vi "Autonomous Independent.vi"() -> ()   [LabVIEW 2012]
doc: "This VI is called when autonomous begins, and will automatically be terminated when autonomous ends. You can carry out timed or sensor driven robot movement independently without needing to return to the caller."
uses:
  <vilib>/Rock Robotics/WPI/Relay/WPI_RelayValue.ctl
  <vilib>/Rock Robotics/WPI/RobotDrive/WPI_RobotDriveGetSetRefNum.vi
  Robot Global Data.vi
panel:
  out "Shooter Speed":T1(ring)
  out "Stop Drive":bool
  out "DT Output":enum16{"Off", "Up", "Down"}(ring)=enum."Down"
  out "BAD Up":bool
  out "DAD Output":T2
  out "Shift Low":bool
  out "Feeder Happy":bool
  out "Auton Done":bool
  out "Shooter Happy":bool
  out "Shoot!":bool
  out "Loop Rate (Hz)":dbl
  out "Delay Switch":u32
  out "Seccond Switch":u32
  out "First Switch":u32
  # "Be sure to right-click and choose Data Operations>>Make Current Value default if you want to save the array values with the VI"
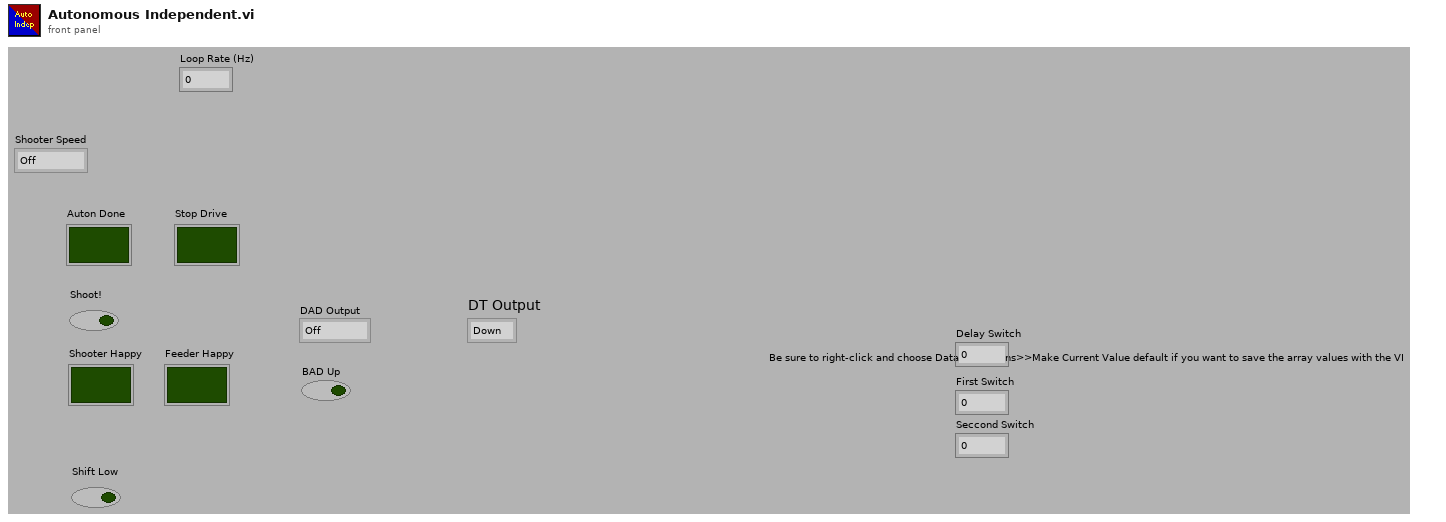
[diagram p1: front panel]
types:
  T1 = enum16{"Off", "Close Pyramid 3pt", "Far Pyramid 3pt", "Feeder Shot"}
  T2 = typedef "WPI_RelayValue.ctl" = enum16{"Off", "On", "Forward", "Reverse"}
  T3 = typedef "WPI_RobotDriveDevRef.ctl" = cluster{"DevStatus":errorcluster, "Motors[]":T4[], "Square Inputs":bool, "Max Output":dbl, "Isochronous":bool}
  T4 = typedef "WPI_MotorControlDeviceRef.ctl" = cluster{"DeviceStatus":errorcluster, "Type":enum16{"PWM", "CAN"}, "PWM":cluster{"Digital Module":T5, "PWM Channel":T6, "DeadBand":T7}, "CAN":cluster{"Device Number":u8, "Control Mode":T8, "Semaphore":T9, "Max Vout":dbl}, "Invert":bool, "TransformRef":T10, "InvTransformRef":T10}
  T5 = typedef "FPGA_TypedefDigitalModule.ctl" = enum16{"Digital Module 1", "Digital Module 2"}
  T6 = typedef "FPGA_DIOPWMChannel.ctl" = enum8{"PWM 1", "PWM 2", "PWM 3", "PWM 4", "PWM 5", "PWM 6", "PWM 7", "PWM 8", "PWM 9", "PWM 10", "Invalid"}
  T7 = typedef "WPI_PWMDeadband.ctl" = cluster{"Name":string, "maxPositivePwm":i32, "minPositivePwm":i32, "centerPwm":i32, "maxNegativePwm":i32, "minNegativePwm":i32, "angularRange":u16}
  T8 = typedef "WPI_CANJaguar_ControlMode.ctl" = enum8{"Percent VBus", "Current", "Speed", "Position", "Voltage"}
  T9 = typedef "Semaphore RefNum" = refnum<k1>
  T10 = typedef "WPI_PWMTransform_ConPane.ctl" = refnum<vi>
  T11 = typedef "WPI_GyroDevRef.ctl" = cluster{"DevStatus":errorcluster, "Analog Module":T12, "Analog Channel":T13, "Offset":dbl, "Gain (VoltsPerDegree/Second)":dbl}
  T12 = typedef "FPGA_TypedefAnalogModule.ctl" = enum16{"Analog Module 1", "Analog Module 2"}
  T13 = typedef "FPGA_AIChannel.ctl" = enum8{"AI 1", "AI 2", "AI 3", "AI 4", "AI 5", "AI 6", "AI 7", "AI 8", "Invalid"}
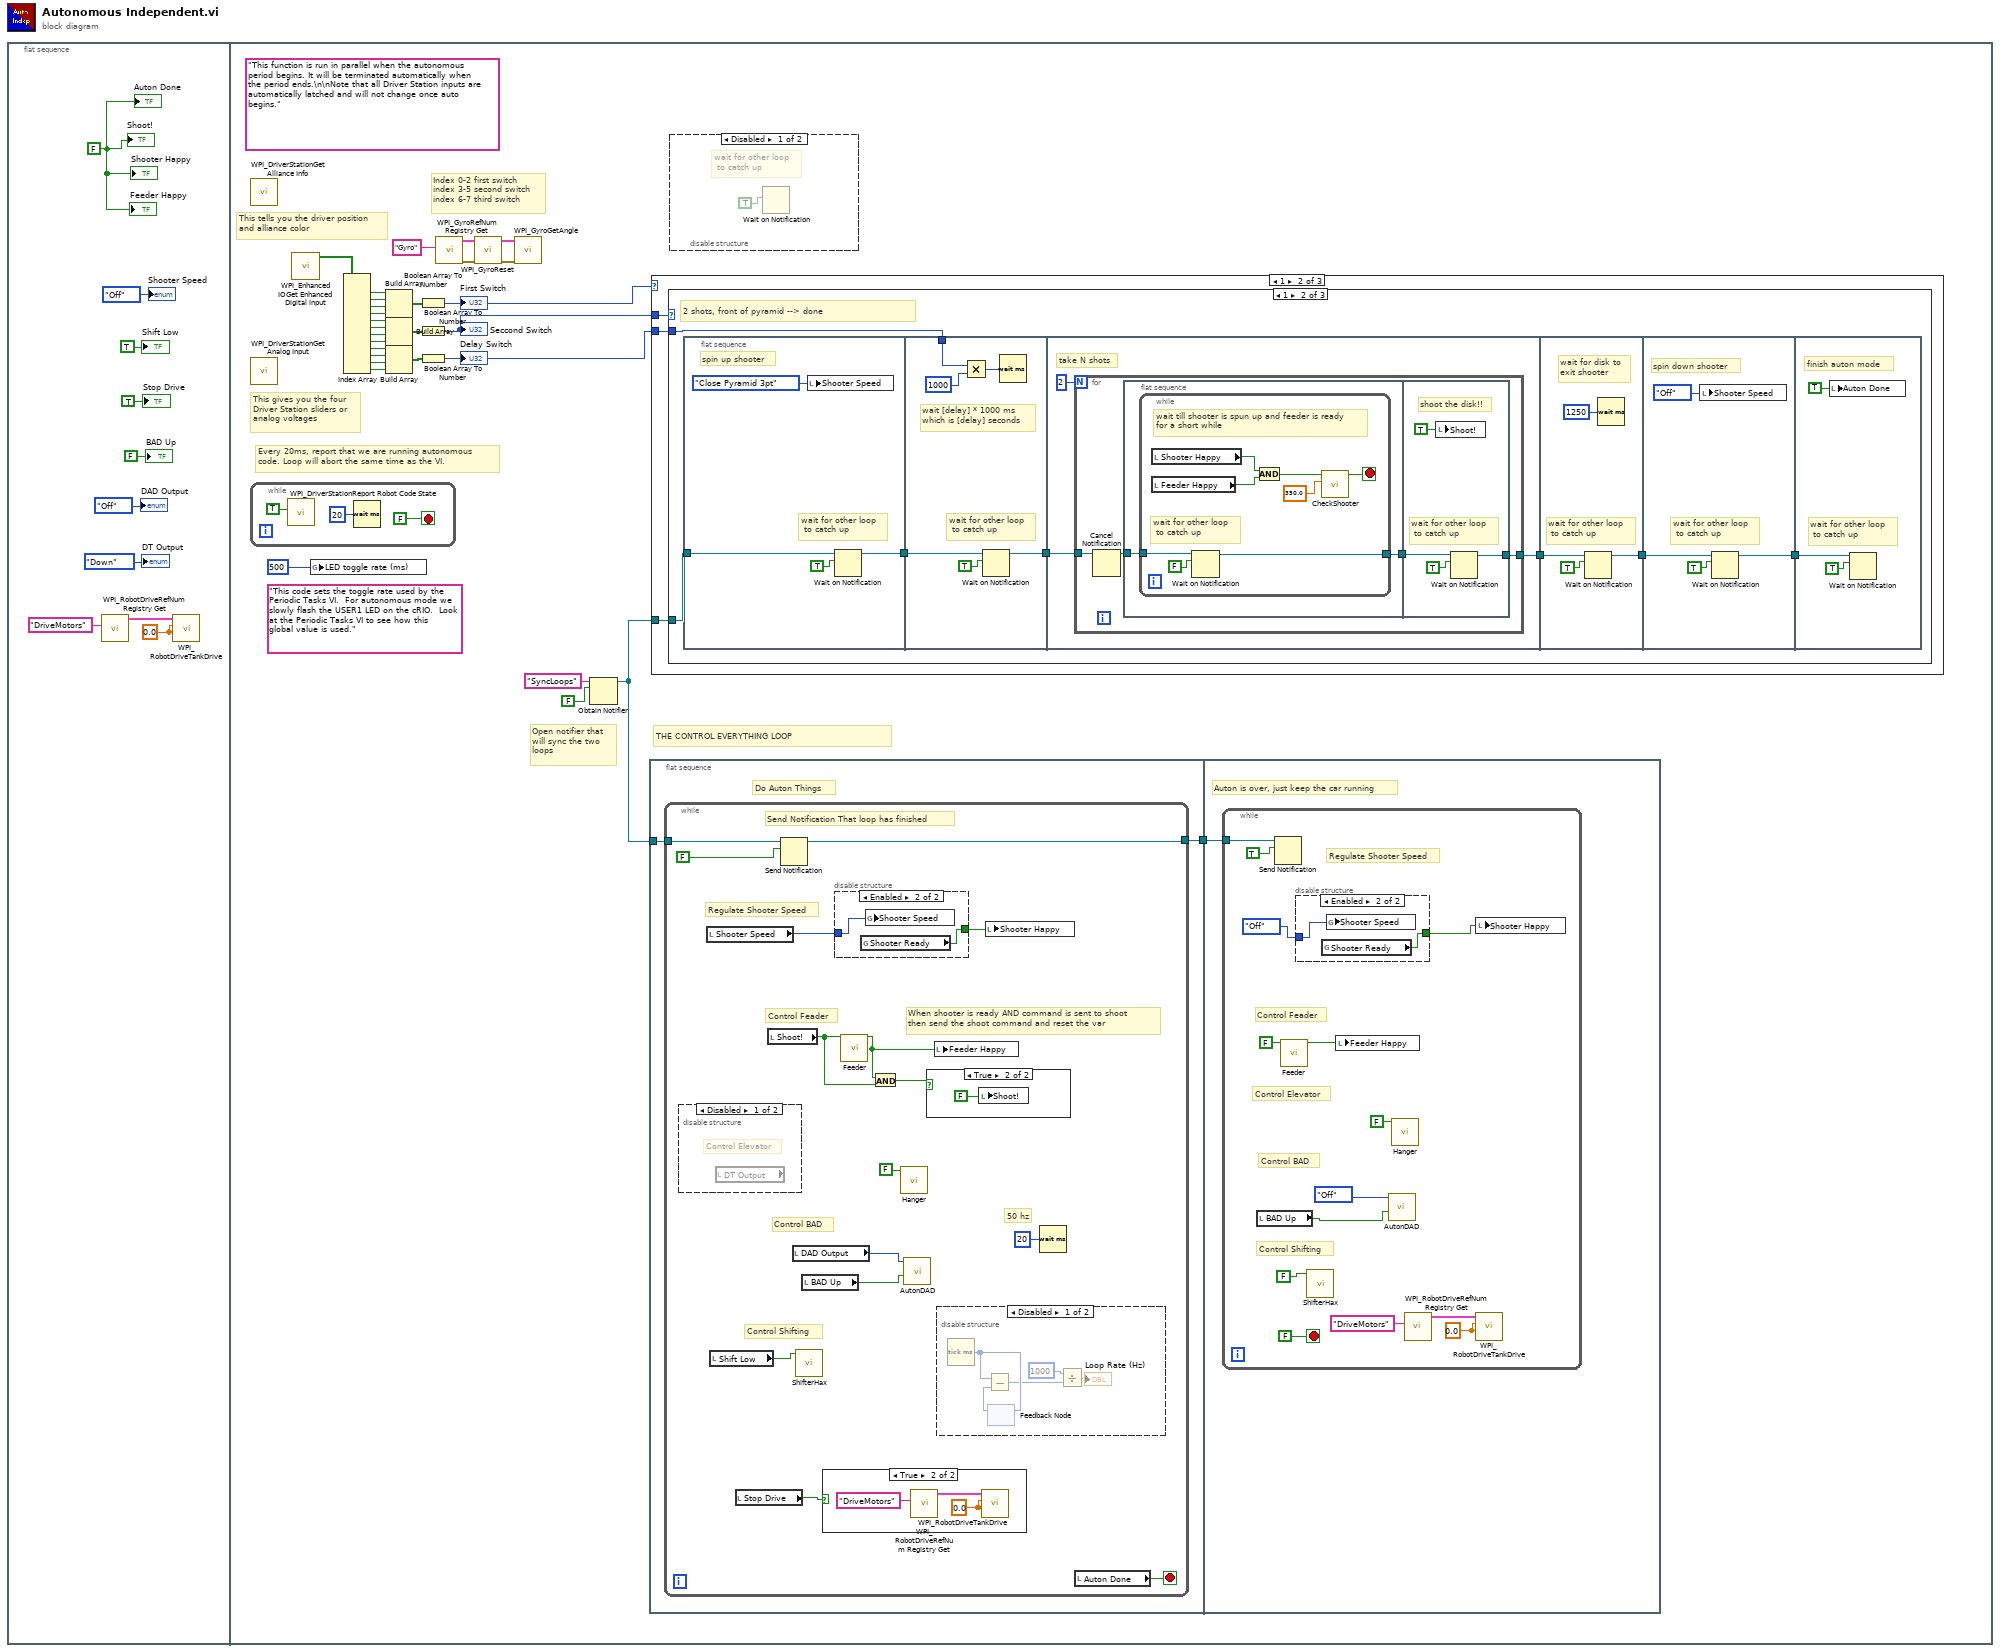
[diagram p0: block diagram]
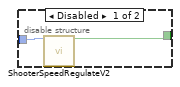
[diagram p3: hidden frame]
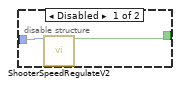
[diagram p8: hidden frame]
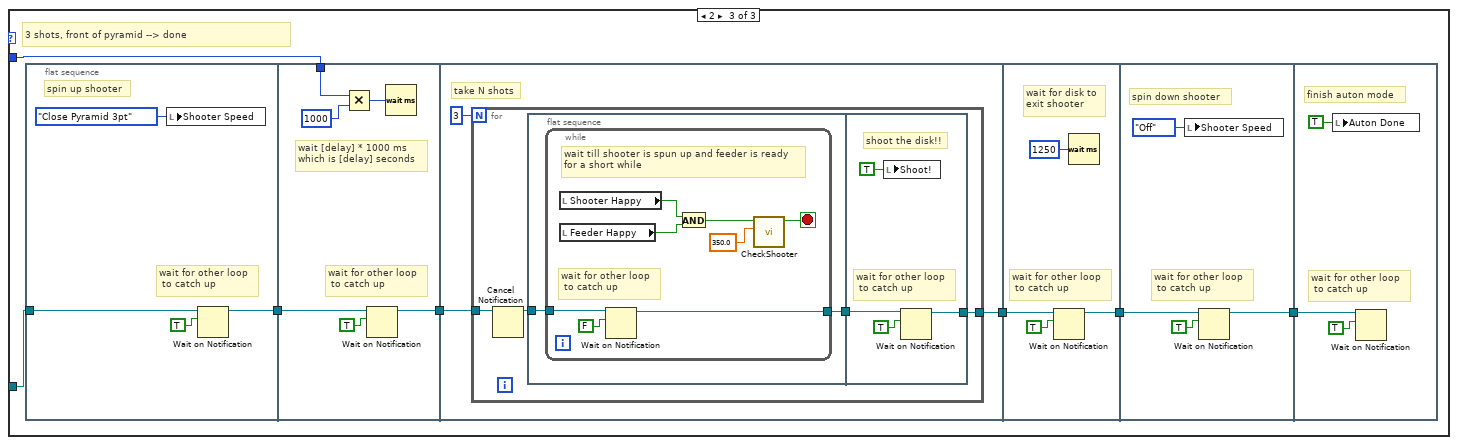
[diagram p11: hidden frame]
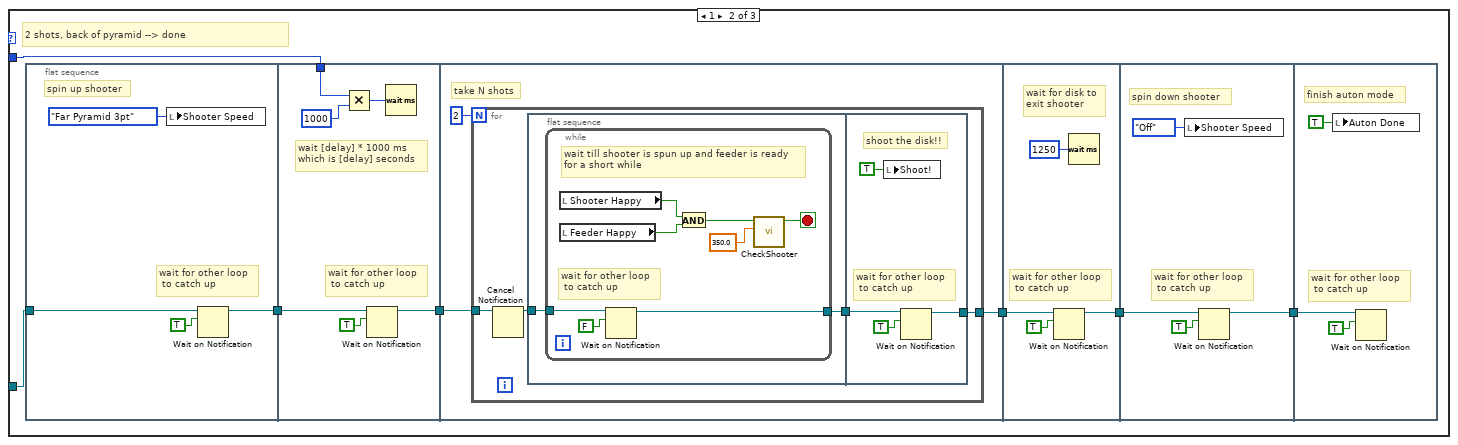
[diagram p13: hidden frame]
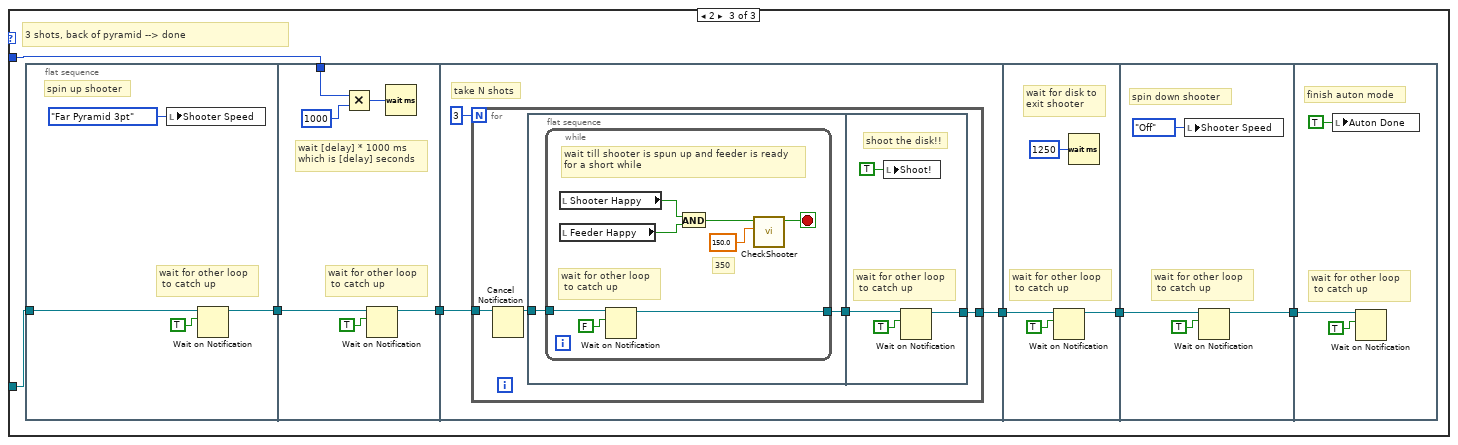
[diagram p14: hidden frame]
diagram:
  n1 = flat-sequence {
    frame #0 {
      w3 = 0.0 ("Left axis value")
      w10 = FALSE
      n2 = call <vilib>:"WPI_RobotDriveRefNum Registry Get.vi"("refnum name"="DriveMotors") -> ("RobotDriveDevRef"=w5:T3)  [unwired: 1 in, 9 out]
      n3 = call <vilib>:"WPI_RobotDriveTankDrive.vi"("Right axis value"=w3, "Left axis value"=w3, "RobotDriveDevRef"=w5) -> ()  [unwired: 6 in, 3 out]
      "Feeder Happy" <- w10
      "Shift Low" <- TRUE ("Shift Low")
      "DAD Output" <- WPI_RelayValue."Off" ("DAD Output")
      "BAD Up" <- FALSE ("BAD Up")
      "Stop Drive" <- TRUE ("Stop Drive")
      "Shoot!" <- w10
      "Shooter Happy" <- w10
      "Auton Done" <- w10
      "DT Output" <- enum16{"Off", "Up", "Down"}."Down" ("DT Output")
      "Shooter Speed" <- T1."Off" ("Shooter Speed")
    }
    frame #1 {
      (unwired) "This code sets the toggle rate used by the Periodic Tasks VI.  For autonomous mode we slowly flash the USER1 LED on the cRIO.  Look at the Periodic Tasks VI to see how this global value is used."
      (unwired) "This function is run in parallel when the autonomous period begins. It will be terminated automatically when the period ends.\n\nNote that all Driver Station inputs are automatically latched and will not change once auto begins."
      # "THE CONTROL EVERYTHING LOOP"
      # "Index 0-2 first switch\nindex 3-5 second switch\nindex 6-7 third switch"
      # "Open notifier that\nwill sync the two\nloops"
      # "Every 20ms, report that we are running autonomous\ncode. Loop will abort the same time as the VI."
      # "This tells you the driver position\nand alliance color"
      # "This gives you the four\nDriver Station sliders or\nanalog voltages"
      n4 = call <vilib>:"WPI_DriverStationGet Alliance Info.vi"() -> ()  [unwired: 12 out]
      n5 = call <vilib>:"WPI_DriverStationGet Analog Input.vi"() -> ()  [unwired: 12 out]
      n6 = while {
        stop <- FALSE stop-if-true
        n7 = call <vilib>:"WPI_DriverStationReport Robot Code State.vi"("Autonomous"=TRUE) -> ()  [unwired: 10 in, 1 out]
        n8 = Wait (ms)(milliseconds to wait=u32 20) -> ()  [unwired: 1 out]
      }
      n9 = call <vilib>:"WPI_Enhanced IOGet Enhanced Digital Input.vi"() -> ("Digital Input [1-16]"=w15:bool[])  [unwired: 10 in, 1 out]
      n10 = global write "Robot Global Data.vi" "LED toggle rate (ms)"(u32 500 ("LED ms toggle rate")) -> ()
      n11 = Index Array(array=w15) -> (element #1=w35:bool, element #2=w34:bool, element #3=w33:bool, element #4=w21:bool, element #5=w32:bool, element #6=w31:bool, element #7=w23:bool, element #8=w22:bool, element #9=w20:bool, element #10=w19:bool, element #11=w18:bool, element #12=w17:bool)  [unwired: 12 in]
      n12 = Build Array(w35, w34, w33, w21) -> (w29:bool[])
      n13 = Build Array(w32, w31, w23, w22) -> (w30:bool[])
      n14 = Build Array(w20, w19, w18, w17) -> (w16:bool[])
      n15 = Boolean Array To Number(Boolean array=w29) -> (number=w14:u32)
      "First Switch" <- w14
      n16 = Boolean Array To Number(Boolean array=w30) -> (number=w13:u32)
      "Seccond Switch" <- w13
      n17 = Boolean Array To Number(Boolean array=w16) -> (number=w11:u32)
      "Delay Switch" <- w11
      n18 = call <vilib>:"WPI_GyroRefNum Registry Get.vi"("refnum name"="Gyro") -> ("error out"=w24:errorcluster, "GyroDevRef"=w25:T11)  [unwired: 9 in]
      n19 = call <vilib>:"WPI_GyroReset.vi"("error in (no error)"=w24, "GyroDevRef"=w25) -> ("error out"=w27:errorcluster, "GyroDevRef"=w26:T11)  [unwired: 8 in]
      n20 = call <vilib>:"WPI_GyroGetAngle.vi"("error in (no error)"=w27, "GyroDevRef"=w26) -> ()  [unwired: 6 in, 4 out]
      n21 = Obtain Notifier(name (unnamed)="SyncLoops", notification data type=FALSE) -> (notifier out=w12:refnum<notifier>)  [unwired: 2 in, 2 out]
      n22 = flat-sequence {
        tunnel: w12 -> [w43]
        tunnel: [w42] -> w39
        tunnel: w39 -> [w72]
        frame #0 {
          # "Do Auton Things"
          n23 = while {
            tunnel: w43 -> [w56]
            tunnel: [w52] -> w42
            stop <- w58 stop-if-true
            # "Regulate Shooter Speed"
            # "50 hz"
            # "Control BAD"
            # "Control Shifting"
            # "When shooter is ready AND command is sent to shoot\nthen send the shoot command and reset the var"
            # "Control Feader"
            # "Send Notification That loop has finished"
            n24 = disable-structure shown="Disabled" {
              frame Disabled {
                # "Control Elevator"
                n25 = local read "DT Output"() -> ()  [unwired: 1 out]
              }
              frame Enabled {
              }
            }
            n26 = local read "Shooter Speed"() -> (w45:T1)
            n27 = local read "Shift Low"() -> (w46:bool)
            n28 = local read "Stop Drive"() -> (w50:bool)
            n29 = local read "Shoot!"() -> (w55:bool)
            n30 = Send Notification(notification=FALSE, notifier=w56) -> (notifier out=w52:refnum<notifier>)  [unwired: 1 in, 1 out]
            n31 = local read "DAD Output"() -> (w48:T2)
            n32 = call "ShifterHax.vi"("Shift low?"=w46) -> ()  [unwired: 11 in]
            n33 = local read "BAD Up"() -> (w49:bool)
            n34 = case shown="True" w50 {
              frame False {
              }
              frame True {
                w65 = 0.0 ("Left axis value")
                n35 = call <vilib>:"WPI_RobotDriveRefNum Registry Get.vi"("refnum name"="DriveMotors") -> ("RobotDriveDevRef"=w63:T3)  [unwired: 1 in, 9 out]
                n36 = call <vilib>:"WPI_RobotDriveTankDrive.vi"("Right axis value"=w65, "Left axis value"=w65, "RobotDriveDevRef"=w63) -> ()  [unwired: 6 in, 3 out]
              }
            }
            n37 = disable-structure shown="Enabled" {
              disable-tunnel: [w60 w61] -> w47
              disable-tunnel: w45 -> [w59 w62]
              frame Disabled {
                n38 = call "ShooterSpeedRegulateV2.vi"("Shooter Speed"=w59) -> ("ALL GOOD"=w60:bool)  [unwired: 13 in, 1 out]
              }
              frame Enabled {
                n39 = global read "Robot Global Data.vi" "Shooter Ready"() -> (w61:bool)
                n40 = global write "Robot Global Data.vi" "Shooter Speed"(w62) -> ()
              }
            }
            n41 = call "Feeder.vi"("SHOOT Button"=w55) -> ("Ready To Shoot?"=w53:bool)  [unwired: 10 in]
            n42 = And(x=w53, y=w55) -> (x .and. y?=w54:bool)
            n43 = call "Hanger.vi"("Hanger Up"=FALSE) -> ()  [unwired: 10 in, 1 out]
            n44 = call "AutonDAD.vi"("BAD UP"=w49, "BAD Output"=w48) -> ()  [unwired: 10 in]
            n45 = case shown="True" w54 {
              frame False {
              }
              frame True {
                n46 = local write "Shoot!"(FALSE) -> ()
              }
            }
            n47 = local write "Feeder Happy"(w53) -> ()
            n48 = disable-structure shown="Disabled" {
              frame Disabled {
                n49 = Tick Count (ms)() -> (millisecond timer value=w70:u32)
                n50 = feedback #1() -> (w69:u32)  [unwired: 1 in]
                n51 = Subtract(x=w70, y=w69) -> (x-y=w67:u32)
                n52 = feedback-in #1(w70) -> ()
                n53 = Divide(x=1000, y=w67) -> (x/y=→"Loop Rate (Hz)":dbl)
              }
              frame Enabled {
              }
            }
            n54 = local write "Shooter Happy"(w47) -> ()
            n55 = Wait (ms)(milliseconds to wait=u32 20) -> ()  [unwired: 1 out]
            n56 = local read "Auton Done"() -> (w58:bool)
          }
        }
        frame #1 {
          # "Auton is over, just keep the car running"
          n57 = while {
            tunnel: w72 -> [w76]
            stop <- FALSE stop-if-true
            w81 = 0.0 ("Left axis value")
            # "Regulate Shooter Speed"
            # "Control BAD"
            # "Control Shifting"
            # "Control Elevator"
            # "Control Feader"
            n58 = local read "BAD Up"() -> (w79:bool)
            n59 = Send Notification(notification=TRUE, notifier=w76) -> ()  [unwired: 1 in, 2 out]
            n60 = call "Feeder.vi"("SHOOT Button"=FALSE) -> ("Ready To Shoot?"=w85:bool)  [unwired: 10 in]
            n61 = disable-structure shown="Enabled" {
              disable-tunnel: [w88 w89] -> w73
              disable-tunnel: T1."Off" ("Shooter Speed") -> [w87 w90]
              frame Disabled {
                n62 = call "ShooterSpeedRegulateV2.vi"("Shooter Speed"=w87) -> ("ALL GOOD"=w88:bool)  [unwired: 13 in, 1 out]
              }
              frame Enabled {
                n63 = global read "Robot Global Data.vi" "Shooter Ready"() -> (w89:bool)
                n64 = global write "Robot Global Data.vi" "Shooter Speed"(w90) -> ()
              }
            }
            n65 = call "ShifterHax.vi"("Shift low?"=FALSE ("Shifting Button")) -> ()  [unwired: 11 in]
            n66 = local write "Feeder Happy"(w85) -> ()
            n67 = call "AutonDAD.vi"("BAD UP"=w79, "BAD Output"=WPI_RelayValue."Off") -> ()  [unwired: 10 in]
            n68 = call "Hanger.vi"("Hanger Up"=FALSE) -> ()  [unwired: 10 in, 1 out]
            n69 = call <vilib>:"WPI_RobotDriveRefNum Registry Get.vi"("refnum name"="DriveMotors") -> ("RobotDriveDevRef"=w83:T3)  [unwired: 1 in, 9 out]
            n70 = call <vilib>:"WPI_RobotDriveTankDrive.vi"("Right axis value"=w81, "Left axis value"=w81, "RobotDriveDevRef"=w83) -> ()  [unwired: 6 in, 3 out]
            n71 = local write "Shooter Happy"(w73) -> ()
          }
        }
      }
      n72 = case shown="1" w14 {
        tunnel: w13 -> [_ w93 w194]
        tunnel: w12 -> [_ w92 w193]
        tunnel: w11 -> [_ w91 w192]
        frame 0, Default {
          # "do nothing"
        }
        frame 1 {
          n73 = case shown="1" w93 {
            tunnel: w92 -> [_ w97 w146]
            tunnel: w91 -> [_ w100 w149]
            frame 0, Default {
              # "do nothing"
            }
            frame 1 {
              # "2 shots, front of pyramid --> done"
              n74 = flat-sequence {
                tunnel: [w103] -> w99
                tunnel: w97 -> [w102]
                tunnel: w100 -> [w108]
                tunnel: w99 -> [w106]
                tunnel: [w105] -> w98
                tunnel: w98 -> [w112]
                tunnel: [w111] -> w94
                tunnel: [w133] -> w95
                tunnel: w94 -> [w132]
                tunnel: [w138] -> w96
                tunnel: w95 -> [w137]
                tunnel: w96 -> [w140]
                frame #0 {
                  # "wait for other loop\n to catch up"
                  # "spin up shooter"
                  n75 = local write "Shooter Speed"(T1."Close Pyramid 3pt" ("Shooter Speed")) -> ()
                  n76 = Wait on Notification(notifier=w102, ignore previous (F)=TRUE) -> (notifier out=w103:refnum<notifier>)  [unwired: 2 in, 3 out]
                }
                frame #1 {
                  # "wait for other loop\n to catch up"
                  # "wait [delay] * 1000 ms\nwhich is [delay] seconds"
                  n77 = Multiply(x=w108, y=1000) -> (x*y=w110:u32)
                  n78 = Wait on Notification(notifier=w106, ignore previous (F)=TRUE) -> (notifier out=w105:refnum<notifier>)  [unwired: 2 in, 3 out]
                  n79 = Wait (ms)(milliseconds to wait=w110) -> ()  [unwired: 1 out]
                }
                frame #2 {
                  # "take N shots"
                  n80 = for {
                    N: 2 -> [_]
                    tunnel: w112 -> [w116]
                    tunnel: [w114] -> w111
                    n81 = Cancel Notification(0:w116) -> (8:w117:refnum<notifier>)  [unwired: 1 in, 2 out]
                    n82 = flat-sequence {
                      tunnel: w117 -> [w119]
                      tunnel: [w118] -> w115
                      tunnel: w115 -> [w129]
                      tunnel: [w128] -> w114
                      frame #0 {
                        n83 = while {
                          tunnel: w119 -> [w121]
                          tunnel: [w120] -> w118
                          stop <- w123 stop-if-true
                          # "wait for other loop\n to catch up"
                          # "wait till shooter is spun up and feeder is ready\nfor a short while"
                          n84 = local read "Shooter Happy"() -> (w126:bool)
                          n85 = local read "Feeder Happy"() -> (w125:bool)
                          n86 = Wait on Notification(notifier=w121, ignore previous (F)=FALSE) -> (notifier out=w120:refnum<notifier>)  [unwired: 2 in, 3 out]
                          n87 = And(x=w126, y=w125) -> (x .and. y?=w124:bool)
                          n88 = call "CheckShooter.vi"("Time for happy (ms)"=350.0, "Shooter Good?"=w124) -> ("Good to shoot"=w123:bool)  [unwired: 9 in]
                        }
                      }
                      frame #1 {
                        # "wait for other loop\n to catch up"
                        # "shoot the disk!!"
                        n89 = local write "Shoot!"(TRUE ("Shoot!")) -> ()
                        n90 = Wait on Notification(notifier=w129, ignore previous (F)=TRUE) -> (notifier out=w128:refnum<notifier>)  [unwired: 2 in, 3 out]
                      }
                    }
                  }
                }
                frame #3 {
                  # "wait for other loop\n to catch up"
                  # "wait for disk to\nexit shooter"
                  n91 = Wait on Notification(notifier=w132, ignore previous (F)=TRUE) -> (notifier out=w133:refnum<notifier>)  [unwired: 2 in, 3 out]
                  n92 = Wait (ms)(milliseconds to wait=u32 1250) -> ()  [unwired: 1 out]
                }
                frame #4 {
                  # "wait for other loop\n to catch up"
                  # "spin down shooter"
                  n93 = local write "Shooter Speed"(T1."Off" ("Shooter Speed")) -> ()
                  n94 = Wait on Notification(notifier=w137, ignore previous (F)=TRUE) -> (notifier out=w138:refnum<notifier>)  [unwired: 2 in, 3 out]
                }
                frame #5 {
                  # "wait for other loop\n to catch up"
                  # "finish auton mode"
                  n95 = local write "Auton Done"(TRUE ("Auton Done")) -> ()
                  n96 = Wait on Notification(notifier=w140, ignore previous (F)=TRUE) -> ()  [unwired: 2 in, 4 out]
                }
              }
            }
            frame 2 {
              # "3 shots, front of pyramid --> done"
              n97 = flat-sequence {
                tunnel: [w152] -> w148
                tunnel: w146 -> [w151]
                tunnel: w149 -> [w157]
                tunnel: w148 -> [w155]
                tunnel: [w154] -> w147
                tunnel: w147 -> [w161]
                tunnel: [w160] -> w143
                tunnel: [w182] -> w144
                tunnel: w143 -> [w181]
                tunnel: [w187] -> w145
                tunnel: w144 -> [w186]
                tunnel: w145 -> [w189]
                frame #0 {
                  # "wait for other loop\n to catch up"
                  # "spin up shooter"
                  n98 = local write "Shooter Speed"(T1."Close Pyramid 3pt" ("Shooter Speed")) -> ()
                  n99 = Wait on Notification(notifier=w151, ignore previous (F)=TRUE) -> (notifier out=w152:refnum<notifier>)  [unwired: 2 in, 3 out]
                }
                frame #1 {
                  # "wait for other loop\n to catch up"
                  # "wait [delay] * 1000 ms\nwhich is [delay] seconds"
                  n100 = Multiply(x=w157, y=1000) -> (x*y=w159:u32)
                  n101 = Wait on Notification(notifier=w155, ignore previous (F)=TRUE) -> (notifier out=w154:refnum<notifier>)  [unwired: 2 in, 3 out]
                  n102 = Wait (ms)(milliseconds to wait=w159) -> ()  [unwired: 1 out]
                }
                frame #2 {
                  # "take N shots"
                  n103 = for {
                    N: 3 -> [_]
                    tunnel: w161 -> [w165]
                    tunnel: [w163] -> w160
                    n104 = Cancel Notification(0:w165) -> (8:w166:refnum<notifier>)  [unwired: 1 in, 2 out]
                    n105 = flat-sequence {
                      tunnel: w166 -> [w168]
                      tunnel: [w167] -> w164
                      tunnel: w164 -> [w178]
                      tunnel: [w177] -> w163
                      frame #0 {
                        n106 = while {
                          tunnel: w168 -> [w170]
                          tunnel: [w169] -> w167
                          stop <- w172 stop-if-true
                          # "wait for other loop\n to catch up"
                          # "wait till shooter is spun up and feeder is ready\nfor a short while"
                          n107 = local read "Shooter Happy"() -> (w175:bool)
                          n108 = local read "Feeder Happy"() -> (w174:bool)
                          n109 = Wait on Notification(notifier=w170, ignore previous (F)=FALSE) -> (notifier out=w169:refnum<notifier>)  [unwired: 2 in, 3 out]
                          n110 = And(x=w175, y=w174) -> (x .and. y?=w173:bool)
                          n111 = call "CheckShooter.vi"("Time for happy (ms)"=350.0, "Shooter Good?"=w173) -> ("Good to shoot"=w172:bool)  [unwired: 9 in]
                        }
                      }
                      frame #1 {
                        # "wait for other loop\n to catch up"
                        # "shoot the disk!!"
                        n112 = local write "Shoot!"(TRUE ("Shoot!")) -> ()
                        n113 = Wait on Notification(notifier=w178, ignore previous (F)=TRUE) -> (notifier out=w177:refnum<notifier>)  [unwired: 2 in, 3 out]
                      }
                    }
                  }
                }
                frame #3 {
                  # "wait for other loop\n to catch up"
                  # "wait for disk to\nexit shooter"
                  n114 = Wait on Notification(notifier=w181, ignore previous (F)=TRUE) -> (notifier out=w182:refnum<notifier>)  [unwired: 2 in, 3 out]
                  n115 = Wait (ms)(milliseconds to wait=u32 1250) -> ()  [unwired: 1 out]
                }
                frame #4 {
                  # "wait for other loop\n to catch up"
                  # "spin down shooter"
                  n116 = local write "Shooter Speed"(T1."Off" ("Shooter Speed")) -> ()
                  n117 = Wait on Notification(notifier=w186, ignore previous (F)=TRUE) -> (notifier out=w187:refnum<notifier>)  [unwired: 2 in, 3 out]
                }
                frame #5 {
                  # "wait for other loop\n to catch up"
                  # "finish auton mode"
                  n118 = local write "Auton Done"(TRUE ("Auton Done")) -> ()
                  n119 = Wait on Notification(notifier=w189, ignore previous (F)=TRUE) -> ()  [unwired: 2 in, 4 out]
                }
              }
            }
          }
        }
        frame 2 {
          n120 = case shown="0, Default" w194 {
            tunnel: w193 -> [_ w198 w247]
            tunnel: w192 -> [_ w201 w250]
            frame 0, Default {
              # "do nothing"
            }
            frame 1 {
              # "2 shots, back of pyramid --> done"
              n121 = flat-sequence {
                tunnel: [w204] -> w200
                tunnel: w198 -> [w203]
                tunnel: w201 -> [w209]
                tunnel: w200 -> [w207]
                tunnel: [w206] -> w199
                tunnel: w199 -> [w213]
                tunnel: [w212] -> w195
                tunnel: [w234] -> w196
                tunnel: w195 -> [w233]
                tunnel: [w239] -> w197
                tunnel: w196 -> [w238]
                tunnel: w197 -> [w241]
                frame #0 {
                  # "wait for other loop\n to catch up"
                  # "spin up shooter"
                  n122 = local write "Shooter Speed"(T1."Far Pyramid 3pt" ("Shooter Speed")) -> ()
                  n123 = Wait on Notification(notifier=w203, ignore previous (F)=TRUE) -> (notifier out=w204:refnum<notifier>)  [unwired: 2 in, 3 out]
                }
                frame #1 {
                  # "wait for other loop\n to catch up"
                  # "wait [delay] * 1000 ms\nwhich is [delay] seconds"
                  n124 = Multiply(x=w209, y=1000) -> (x*y=w211:u32)
                  n125 = Wait on Notification(notifier=w207, ignore previous (F)=TRUE) -> (notifier out=w206:refnum<notifier>)  [unwired: 2 in, 3 out]
                  n126 = Wait (ms)(milliseconds to wait=w211) -> ()  [unwired: 1 out]
                }
                frame #2 {
                  # "take N shots"
                  n127 = for {
                    N: 2 -> [_]
                    tunnel: w213 -> [w217]
                    tunnel: [w215] -> w212
                    n128 = Cancel Notification(0:w217) -> (8:w218:refnum<notifier>)  [unwired: 1 in, 2 out]
                    n129 = flat-sequence {
                      tunnel: w218 -> [w220]
                      tunnel: [w219] -> w216
                      tunnel: w216 -> [w230]
                      tunnel: [w229] -> w215
                      frame #0 {
                        n130 = while {
                          tunnel: w220 -> [w222]
                          tunnel: [w221] -> w219
                          stop <- w224 stop-if-true
                          # "wait for other loop\n to catch up"
                          # "wait till shooter is spun up and feeder is ready\nfor a short while"
                          n131 = local read "Shooter Happy"() -> (w227:bool)
                          n132 = local read "Feeder Happy"() -> (w226:bool)
                          n133 = Wait on Notification(notifier=w222, ignore previous (F)=FALSE) -> (notifier out=w221:refnum<notifier>)  [unwired: 2 in, 3 out]
                          n134 = And(x=w227, y=w226) -> (x .and. y?=w225:bool)
                          n135 = call "CheckShooter.vi"("Time for happy (ms)"=350.0, "Shooter Good?"=w225) -> ("Good to shoot"=w224:bool)  [unwired: 9 in]
                        }
                      }
                      frame #1 {
                        # "wait for other loop\n to catch up"
                        # "shoot the disk!!"
                        n136 = local write "Shoot!"(TRUE ("Shoot!")) -> ()
                        n137 = Wait on Notification(notifier=w230, ignore previous (F)=TRUE) -> (notifier out=w229:refnum<notifier>)  [unwired: 2 in, 3 out]
                      }
                    }
                  }
                }
                frame #3 {
                  # "wait for other loop\n to catch up"
                  # "wait for disk to\nexit shooter"
                  n138 = Wait on Notification(notifier=w233, ignore previous (F)=TRUE) -> (notifier out=w234:refnum<notifier>)  [unwired: 2 in, 3 out]
                  n139 = Wait (ms)(milliseconds to wait=u32 1250) -> ()  [unwired: 1 out]
                }
                frame #4 {
                  # "wait for other loop\n to catch up"
                  # "spin down shooter"
                  n140 = local write "Shooter Speed"(T1."Off" ("Shooter Speed")) -> ()
                  n141 = Wait on Notification(notifier=w238, ignore previous (F)=TRUE) -> (notifier out=w239:refnum<notifier>)  [unwired: 2 in, 3 out]
                }
                frame #5 {
                  # "wait for other loop\n to catch up"
                  # "finish auton mode"
                  n142 = local write "Auton Done"(TRUE ("Auton Done")) -> ()
                  n143 = Wait on Notification(notifier=w241, ignore previous (F)=TRUE) -> ()  [unwired: 2 in, 4 out]
                }
              }
            }
            frame 2 {
              # "3 shots, back of pyramid --> done"
              n144 = flat-sequence {
                tunnel: [w253] -> w249
                tunnel: w247 -> [w252]
                tunnel: w250 -> [w258]
                tunnel: w249 -> [w256]
                tunnel: [w255] -> w248
                tunnel: w248 -> [w262]
                tunnel: [w261] -> w244
                tunnel: [w283] -> w245
                tunnel: w244 -> [w282]
                tunnel: [w288] -> w246
                tunnel: w245 -> [w287]
                tunnel: w246 -> [w290]
                frame #0 {
                  # "wait for other loop\n to catch up"
                  # "spin up shooter"
                  n145 = local write "Shooter Speed"(T1."Far Pyramid 3pt" ("Shooter Speed")) -> ()
                  n146 = Wait on Notification(notifier=w252, ignore previous (F)=TRUE) -> (notifier out=w253:refnum<notifier>)  [unwired: 2 in, 3 out]
                }
                frame #1 {
                  # "wait for other loop\n to catch up"
                  # "wait [delay] * 1000 ms\nwhich is [delay] seconds"
                  n147 = Multiply(x=w258, y=1000) -> (x*y=w260:u32)
                  n148 = Wait on Notification(notifier=w256, ignore previous (F)=TRUE) -> (notifier out=w255:refnum<notifier>)  [unwired: 2 in, 3 out]
                  n149 = Wait (ms)(milliseconds to wait=w260) -> ()  [unwired: 1 out]
                }
                frame #2 {
                  # "take N shots"
                  n150 = for {
                    N: 3 -> [_]
                    tunnel: w262 -> [w266]
                    tunnel: [w264] -> w261
                    n151 = Cancel Notification(0:w266) -> (8:w267:refnum<notifier>)  [unwired: 1 in, 2 out]
                    n152 = flat-sequence {
                      tunnel: w267 -> [w269]
                      tunnel: [w268] -> w265
                      tunnel: w265 -> [w279]
                      tunnel: [w278] -> w264
                      frame #0 {
                        n153 = while {
                          tunnel: w269 -> [w271]
                          tunnel: [w270] -> w268
                          stop <- w273 stop-if-true
                          # "350"
                          # "wait for other loop\n to catch up"
                          # "wait till shooter is spun up and feeder is ready\nfor a short while"
                          n154 = local read "Shooter Happy"() -> (w276:bool)
                          n155 = local read "Feeder Happy"() -> (w275:bool)
                          n156 = Wait on Notification(notifier=w271, ignore previous (F)=FALSE) -> (notifier out=w270:refnum<notifier>)  [unwired: 2 in, 3 out]
                          n157 = And(x=w276, y=w275) -> (x .and. y?=w274:bool)
                          n158 = call "CheckShooter.vi"("Time for happy (ms)"=150.0, "Shooter Good?"=w274) -> ("Good to shoot"=w273:bool)  [unwired: 9 in]
                        }
                      }
                      frame #1 {
                        # "wait for other loop\n to catch up"
                        # "shoot the disk!!"
                        n159 = local write "Shoot!"(TRUE ("Shoot!")) -> ()
                        n160 = Wait on Notification(notifier=w279, ignore previous (F)=TRUE) -> (notifier out=w278:refnum<notifier>)  [unwired: 2 in, 3 out]
                      }
                    }
                  }
                }
                frame #3 {
                  # "wait for other loop\n to catch up"
                  # "wait for disk to\nexit shooter"
                  n161 = Wait on Notification(notifier=w282, ignore previous (F)=TRUE) -> (notifier out=w283:refnum<notifier>)  [unwired: 2 in, 3 out]
                  n162 = Wait (ms)(milliseconds to wait=u32 1250) -> ()  [unwired: 1 out]
                }
                frame #4 {
                  # "wait for other loop\n to catch up"
                  # "spin down shooter"
                  n163 = local write "Shooter Speed"(T1."Off" ("Shooter Speed")) -> ()
                  n164 = Wait on Notification(notifier=w287, ignore previous (F)=TRUE) -> (notifier out=w288:refnum<notifier>)  [unwired: 2 in, 3 out]
                }
                frame #5 {
                  # "wait for other loop\n to catch up"
                  # "finish auton mode"
                  n165 = local write "Auton Done"(TRUE ("Auton Done")) -> ()
                  n166 = Wait on Notification(notifier=w290, ignore previous (F)=TRUE) -> ()  [unwired: 2 in, 4 out]
                }
              }
            }
          }
        }
      }
      n167 = disable-structure shown="Disabled" {
        frame Disabled {
          # "wait for other loop\n to catch up"
          n168 = Wait on Notification(ignore previous (F)=TRUE) -> (notifier=w41:refnum<notifier>)  [unwired: 2 in, 4 out]
        }
        frame Enabled {
        }
      }
    }
  }
